vi "JV SN2.vi"(10 "reference":refnum<vi>, 11 "Boolean in":refnum<vi>) -> ()   [LabVIEW 2018]
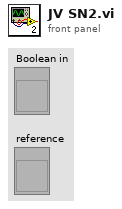
[diagram p1: front panel]
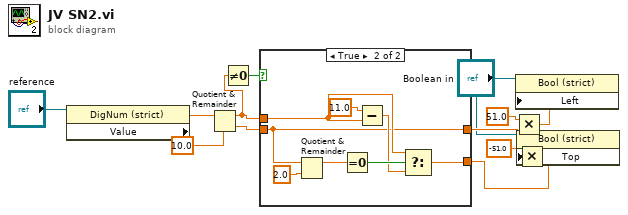
[diagram p0: block diagram]
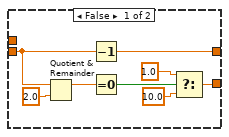
[diagram p2: hidden frame]
diagram:
  n1 = property class="DigNum (strict)"(reference="reference") -> ("Value"=w6:dbl)  [unwired: 1 in, 2 out]
  n2 = Quotient & Remainder(x=w6, y=10.0) -> (x-y*floor(x/y)=w11:dbl, floor(x/y)=w10:dbl)
  n3 = Not Equal To 0?(x=w11) -> (x != 0?=w9:bool)
  n4 = case shown="True" w9 {
    tunnel: [w15 w23] -> w12
    tunnel: w11 -> [_ w24]
    tunnel: w10 -> [w16 w23]
    tunnel: [w14 w22] -> w13
    frame False {
      n5 = Quotient & Remainder(x=w16, y=2.0) -> (x-y*floor(x/y)=w20:dbl)  [unwired: 1 out]
      n6 = Decrement(x=w16) -> (x-1=w15:dbl)
      n7 = Equal To 0?(x=w20) -> (x = 0?=w19:bool)
      n8 = Select(t=1.0, s=w19, f=10.0) -> (s? t:f=w14:dbl)
    }
    frame True {
      n9 = Quotient & Remainder(x=w23, y=2.0) -> (x-y*floor(x/y)=w25:dbl)  [unwired: 1 out]
      n10 = Equal To 0?(x=w25) -> (x = 0?=w28:bool)
      n11 = Subtract(x=11.0, y=w24) -> (x-y=w26:dbl)
      n12 = Select(t=w24, s=w28, f=w26) -> (s? t:f=w22:dbl)
    }
  }
  n13 = Multiply(x=51.0, y=w13) -> (x*y=w7:dbl)
  n14 = property on="Property Node" class="Bool (strict)"(reference="Boolean in", "Left"=w7) -> ()  [unwired: 1 in, 2 out]
  n15 = Multiply(x=-51.0, y=w12) -> (x*y=w8:dbl)
  n16 = property on="Property Node" class="Bool (strict)"(reference="Boolean in", "Top"=w8) -> ()  [unwired: 1 in, 2 out]
